vi "集成多参数全参数数据插入.vi"(0 "Tabe Name":string, 1 "data":variant[](array[variant]), 2 "columns外部输入":T1, 3 "错误输入（无错误）":errorcluster, 4 "数据库类型":T2, 5 "Password":string) -> (10 "错误输出":errorcluster)   [LabVIEW 2016]
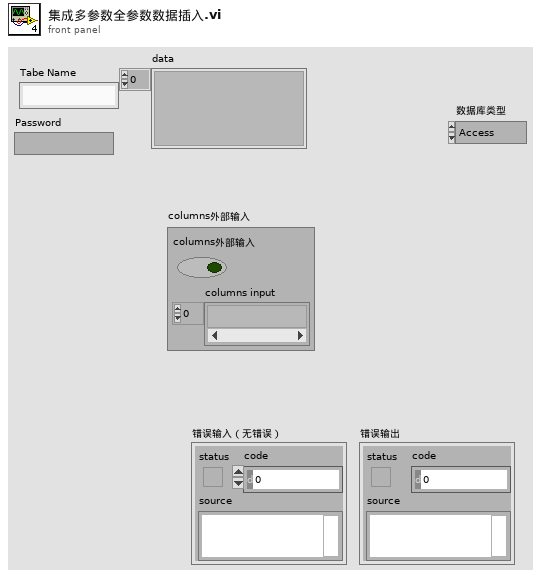
[diagram p1: front panel]
types:
  T1 = cluster{"columns外部输入":bool, "columns input":string[]}
  T2 = typedef "数据库类型.ctl" = enum16{"Access", "SQLite"}
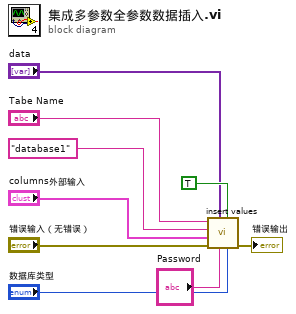
[diagram p0: block diagram]
diagram:
  n1 = call "insert values.vi"("数据库类型"="数据库类型", "是否创建唯一键"=TRUE, "Password"="Password", "data"="data", "错误输入（无错误）"="错误输入（无错误）", "columns外部输入"="columns外部输入", "database"="database1", "Tabe Name"="Tabe Name") -> ("错误输出"=→"错误输出":errorcluster)  [unwired: 3 in]
